vi "SetCalMotor.vi"(7 "LabVIEW Web Service Request":refnum<class "Web Request.lvclass">, 11 "motor":string) -> (3 "result":string)   [LabVIEW 2016]
uses:
  <vilib>/wsapi/Web Request.lvclass
  controls/SwitchStates.ctl
panel:
  # "Use the Web Service Request input terminal to call the VIs on the Web Services palette. Do not remove it from the connector pane unless you don't need access to the palette."
  # "Each additional control wired to the connector pane will be available as an input in the URL. To include an indicator in terminal-mode output (the default setting), it must also be wired to the connector pane."
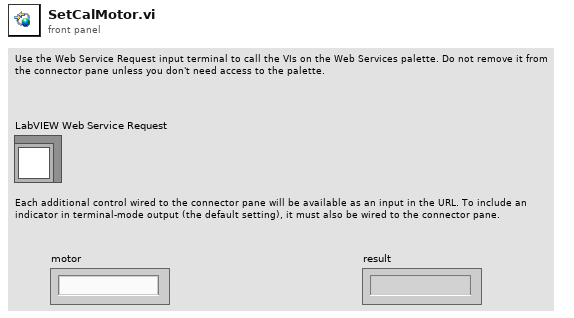
[diagram p1: front panel]
types:
  T1 = typedef "RT-Variables.lvlib/SwitchStates.ctl" = enum16{"Off", "Local", "Remote"}
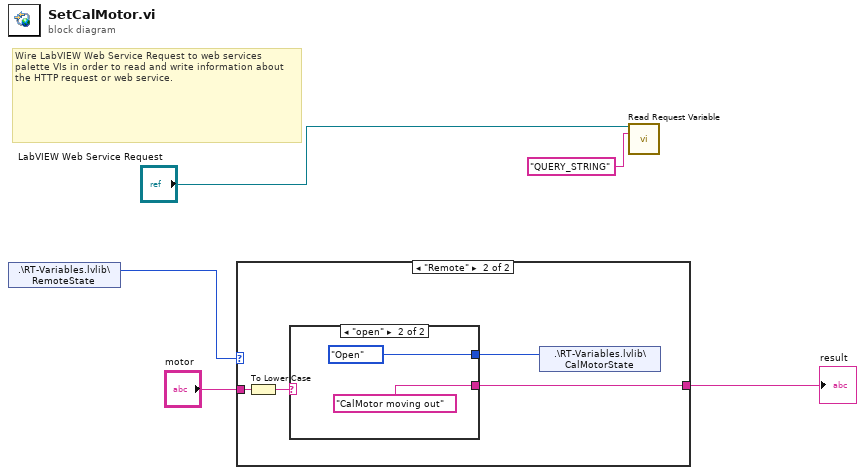
[diagram p0: block diagram]
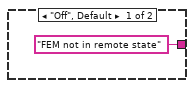
[diagram p2: hidden frame]
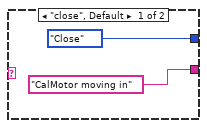
[diagram p3: hidden frame]
diagram:
  # "Wire LabVIEW Web Service Request to web services palette VIs in order to read and write information about the HTTP request or web service."
  n1 = shared-variable ".\\RT-Variables.lvlib\\RemoteState"() -> (w4:T1)  [unwired: 1 in, 1 out]
  n2 = case shown="\"Remote\"" w4 {
    tunnel: "motor" -> [_ w10]
    tunnel: ["FEM not in remote state" w7] -> w3
    frame "Off", Default {
    }
    frame "Remote" {
      n3 = To Lower Case(string=w10) -> (all lower case string=w9:string)
      n4 = case shown="\"open\"" w9 {
        tunnel: [enum16{"Open", "Moving", "Close", "Wait"}."Close" ("CoverState") enum16{"Open", "Moving", "Close", "Wait"}."Open" ("CoverState")] -> w8
        tunnel: ["CalMotor moving in" "CalMotor moving out"] -> w7
        frame "close", Default {
        }
        frame "open" {
        }
      }
      n5 = shared-variable ".\\RT-Variables.lvlib\\CalMotorState"(w8) -> ()  [unwired: 1 in, 1 out]
    }
  }
  "result" <- w3
  n6 = call <vilib>:"Read Request Variable.vi"("LabVIEW Web Service Request"="LabVIEW Web Service Request", "variable name"="QUERY_STRING") -> ()  [unwired: 11 in, 3 out]
